vi "Select Rectangle.vi"(5 "Type":i32, 7 "Tool":i32(ring)=2 items=["None", "Selection Tool", "Point Tool", "Line Tool", "Rectangle Tool", "Oval Tool", "Polygon Tool", "ClosedFreehandTool", "Annulus Tool", "Rotated Rectangle Tool", "Zoom Tool", "Pan Tool", "Polyline Tool", "Freehand Tool"], 8 "Boundary":i16, 9 "Reference Rectangle":i16[][](array[numeric]), 10 "Coordinates":i32[](array[numeric]), 11 "Image In":T1) -> (0 "Height (pixels)":i32, 1 "Width (pixels)":i32, 2 "Selected Reference Rectangle":i16[](array[numeric]), 3 "Image Out":T1)   [LabVIEW 2020]
uses:
  <vilib>/vision/Image Controls.llb/IMAQ Image.ctl
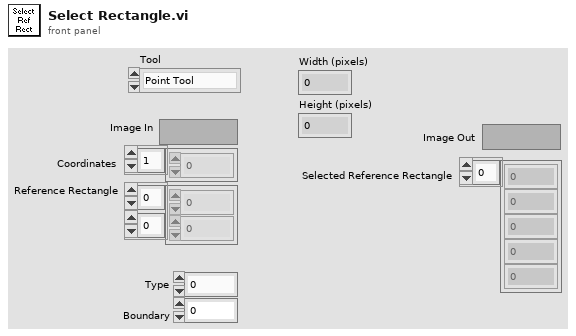
[diagram p1: front panel]
types:
  T1 = typedef "IMAQ Image.ctl" = refnum<image>
  T2 = cluster{"Left":i32, "Top":i32, "Right":i32, "Bottom":i32}
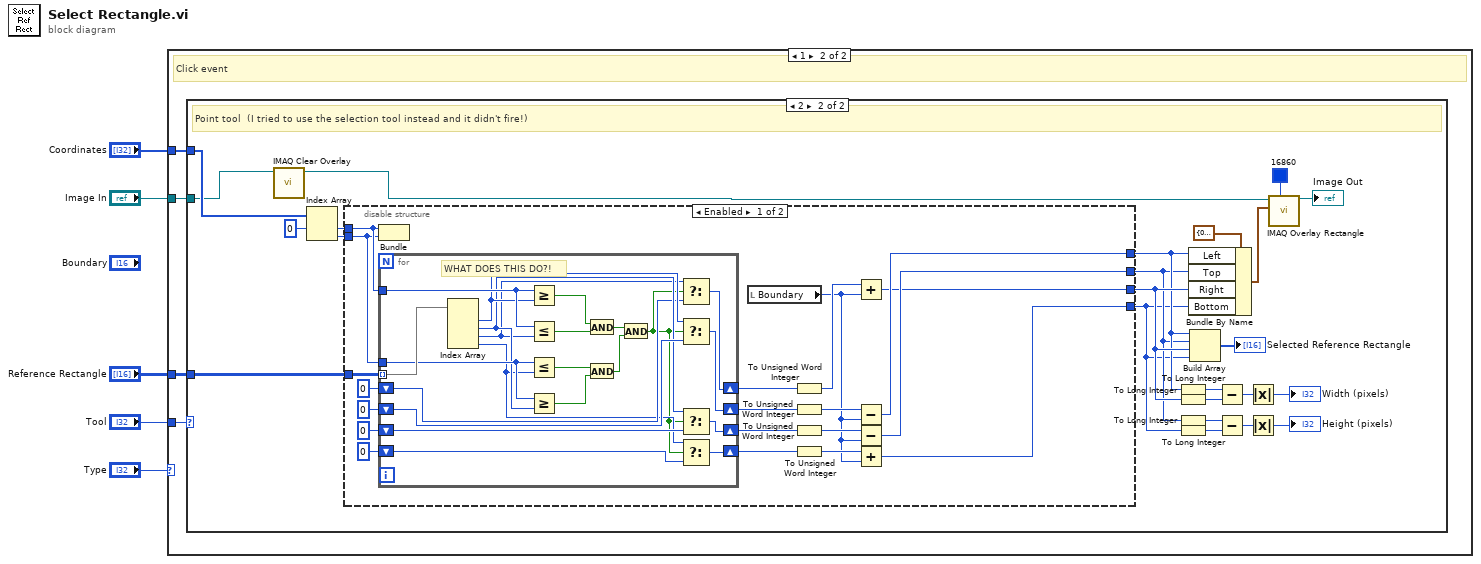
[diagram p0: block diagram]
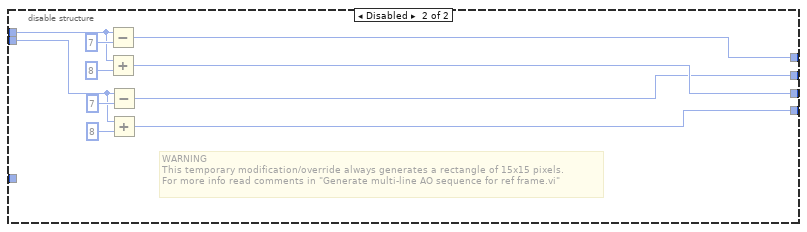
[diagram p4: hidden frame]
diagram:
  n1 = case shown="1" "Type" {
    tunnel: "Tool" -> [_ w9]
    tunnel: "Coordinates" -> [_ w8]
    tunnel: "Image In" -> [_ w7]
    tunnel: "Reference Rectangle" -> [_ w6]
    frame Default {
      # "Any other event"
    }
    frame 1 {
      # "Click event"
      n2 = case shown="2" w9 {
        tunnel: w8 -> [_ w31]
        tunnel: w7 -> [_ w22]
        tunnel: w6 -> [_ w30]
        frame Default {
          # "Any other tool"
        }
        frame 2 {
          # "Point tool  (I tried to use the selection tool instead and it didn't fire!)"
          n3 = call "IMAQ Clear Overlay"("Image"=w22) -> ("Image Out"=w23:T1)  [unwired: 9 in, 1 out]
          n4 = Index Array(array=w31, index #1=0 ("index")) -> (element #1=w29:i32, element #2=w28:i32)  [unwired: 1 in]
          n5 = disable-structure shown="Enabled" {
            disable-tunnel: w30 -> [w53 _]
            disable-tunnel: w29 -> [w52 w83]
            disable-tunnel: w28 -> [w51 w78]
            disable-tunnel: [w37 w84] -> w20
            disable-tunnel: [w36 w77] -> w11
            disable-tunnel: [w35 w81] -> w21
            disable-tunnel: [w34 w76] -> w10
            frame Enabled {
              n6 = Bundle(w52, w51) -> ()  [unwired: 1 in, 1 out]
              n7 = for {
                tunnel: w53 -> [w75] mode=indexing
                tunnel: w52 -> [w74]
                tunnel: w51 -> [w69]
                shift-right: [w66] -> w38
                shift-left: i16 0 -> [w65]
                shift-right: [w62] -> w42
                shift-left: i16 0 ("Numeric") -> [w61]
                shift-right: [w59] -> w44
                shift-left: i16 0 ("Numeric") -> [w58]
                shift-right: [w56] -> w40
                shift-left: i16 0 ("Numeric") -> [w55]
                # "WHAT DOES THIS DO?!"
                n8 = Index Array(array=w75) -> (element #1=w64:i16, element #2=w63:i16, element #3=w60:i16, element #4=w57:i16)  [unwired: 4 in]
                n9 = Greater Or Equal?(x=w74, y=w64) -> (x >= y?=w73:bool)
                n10 = Less Or Equal?(x=w74, y=w60) -> (x <= y?=w72:bool)
                n11 = Less Or Equal?(x=w69, y=w57) -> (x <= y?=w71:bool)
                n12 = Greater Or Equal?(x=w69, y=w63) -> (x >= y?=w70:bool)
                n13 = And(x=w73, y=w72) -> (x .and. y?=w68:bool)
                n14 = And(x=w71, y=w70) -> (x .and. y?=w67:bool)
                n15 = And(x=w68, y=w67) -> (x .and. y?=w54:bool)
                n16 = Select(t=w60, s=w54, f=w58) -> (s? t:f=w59:i16)
                n17 = Select(t=w64, s=w54, f=w65) -> (s? t:f=w66:i16)
                n18 = Select(t=w63, s=w54, f=w61) -> (s? t:f=w62:i16)
                n19 = Select(t=w57, s=w54, f=w55) -> (s? t:f=w56:i16)
              }
              n20 = local read "Boundary"() -> (w39:i16)
              n21 = To Unsigned Word Integer(number=w44) -> (unsigned 16bit integer=w45:u16)
              n22 = To Unsigned Word Integer(number=w38) -> (unsigned 16bit integer=w46:u16)
              n23 = To Unsigned Word Integer(number=w42) -> (unsigned 16bit integer=w43:u16)
              n24 = To Unsigned Word Integer(number=w40) -> (unsigned 16bit integer=w41:u16)
              n25 = Add(x=w45, y=w39) -> (x+y=w35:u16)
              n26 = Subtract(x=w46, y=w39) -> (x-y=w37:u16)
              n27 = Subtract(x=w43, y=w39) -> (x-y=w36:u16)
              n28 = Add(x=w41, y=w39) -> (x+y=w34:u16)
            }
            frame Disabled {
              # "WARNING\nThis temporary modification/override always generates a rectangle of 15x15 pixels.\nFor more info read comments in \"Generate multi-line AO sequence for ref frame.vi\""
              n29 = Subtract(x=w83, y=7) -> (x-y=w84:i32)
              n30 = Add(x=w83, y=8) -> (x+y=w81:i32)
              n31 = Subtract(x=w78, y=7) -> (x-y=w77:i32)
              n32 = Add(x=w78, y=8) -> (x+y=w76:i32)
            }
          }
          n33 = To Long Integer(number=w20) -> (32bit integer=w19:i32)
          n34 = To Long Integer(number=w21) -> (32bit integer=w18:i32)
          n35 = To Long Integer(number=w11) -> (32bit integer=w14:i32)
          n36 = To Long Integer(number=w10) -> (32bit integer=w15:i32)
          n37 = Bundle By Name(cluster=T2 {"Left"=0, "Top"=0, "Right"=0, "Bottom"=0} ("Rectangle"), "Left"=w20, "Top"=w11, "Right"=w21, "Bottom"=w10) -> (w25:T2)
          n38 = Build Array(w20, w11, w21, w10) -> (→"Selected Reference Rectangle":u16[])
          n39 = Subtract(x=w19, y=w18) -> (x-y=w17:i32)
          n40 = Subtract(x=w14, y=w15) -> (x-y=w16:i32)
          n41 = Absolute Value(x=w17) -> (abs(x)=→"Width (pixels)":i32)
          n42 = Absolute Value(x=w16) -> (abs(x)=→"Height (pixels)":i32)
          n43 = call "IMAQ Overlay Rectangle"("Color"=u32 16860 ("Text Color (black)"), "Rectangle"=w25, "Image"=w23) -> ("Image Out"=→"Image Out":T1)  [unwired: 7 in, 1 out]
        }
      }
    }
  }
